vi "Measurement UI.vi"() -> ()   [LabVIEW 2021, in "Load Transient Response_PMIC.lvlib"]
uses:
  Load Transient Response_PMIC.lvlib
panel:
  in  "MeasGraphs":enum32{"LOAD TRANSIENT", "Hidden Controls"}(tab)
  out "LoadCurrentV/STimeGraph":waveform(dbl)(graph) caption="Load Transient"
  out "OutputVoltageV/STimeGraph":waveform(dbl)(graph) caption="Load Transient"
  in  "Load Current v/s Time":string="LOAD CURRENT vs TIME"
  in  "Output Voltage v/s Time":string="LOAD VOLTAGE vs TIME"
  in  "Source resource name":string
  in  "Load resource name":string
  out "dt":dbl
  out "Load voltages":dbl[](array[numeric])
  out "Load currents":dbl[](array[numeric])
  in  "Source transient response":i32(ring)=1042 items=["Slow"=1041, "Normal"=1038, "Fast"=1039, "Custom"=1042]
  in  "Load transient response":i32(ring)=3 items=["Slow"=1041, "Normal"=1038, "Fast"=1039, "Custom"=1042]
  in  "Load current level range":dbl=6.0 caption="CURRENT LEVEL RANGE" format="%#_6pA"
  in  "Load current rising slew rate":dbl=24.0 caption="CURRENT RISING SLEW RATE" format="%#_6pA/us"
  in  "Load current falling slew rate":dbl=24.0 caption="CURRENT FALLING SLEW RATE" format="%#_6pA/us"
  in  "Load configuration":string="Load configuration"
  in  "Source configuration":string="Source configuration"
  in  "Source voltage level":dbl=12.0 caption="VOLTAGE LEVEL" format="%#_6pV"
  in  "Source current limit":dbl=25.0 caption="CURRENT LIMIT" format="%#_6pA"
  in  "PPSResourceName":refnum<k15> caption="RESOURCE NAME"
  in  "Source voltage pole-zero ratio":dbl=2.0 caption="POLE-ZERO RATIO"
  in  "Source voltage gain bandwidth":dbl=2000.0 caption="GAIN BANDWIDTH" format="%#_6pHz"
  in  "Source voltage compensation frequency":dbl=3530.0 caption="COMP. FREQUENCY" format="%#_6pHz"
  in  "Source fast":bool
  in  "Source normal":bool
  in  "Source slow":bool
  in  "Source SourceAdapt":string="Voltage SourceAdapt Parameters"
  in  "Load voltage limit range":dbl=6.0 caption="VOLTAGE LIMIT RANGE" format="%#_6pV"
  in  "Load current set point 1":dbl=4.0 caption="CURRENT SET POINT 1" format="%#_6pA"
  in  "Load current pole-zero ratio":dbl=0.3 caption="POLE-ZERO RATIO"
  in  "Load current gain bandwidth":dbl=14000.0 caption="GAIN BANDWIDTH" format="%#_6pHz"
  in  "Load current compensation frequency":dbl=180000.0 caption="COMP. FREQUENCY" format="%#_6pHz"
  in  "Load sample rate":dbl=1800000.0 caption="SAMPLE RATE" format="%#_6pS/s"
  in  "Load current set point 2":dbl=14.0 caption="CURRENT SET POINT 2" format="%#_6pA"
  in  "ELOADResourceName":refnum<k15> caption="RESOURCE NAME"
  in  "Load fast":bool
  in  "Load normal":bool
  in  "Load slow":bool
  in  "Load SourceAdapt":string="Current SourceAdapt Parameters"
  out "Status":string
  in  "DUT setup time":dbl=1.0 caption="DUT SETUP TIME" format="%#_6ps"
  in  "Level dwell time":dbl=0.001 caption="LEVEL DWELL TIME" format="%#_6ps"
  in  "Measurement settings":string="Measurement settings"
  in  "Nominal output voltage":dbl=3.3 caption="NOMINAL OUTPUT VOLTAGE" format="%#_6pV"
  in  "Mode of operation":T1(ring)=enum."Perform measurement" caption="MODE OF OPERATION"
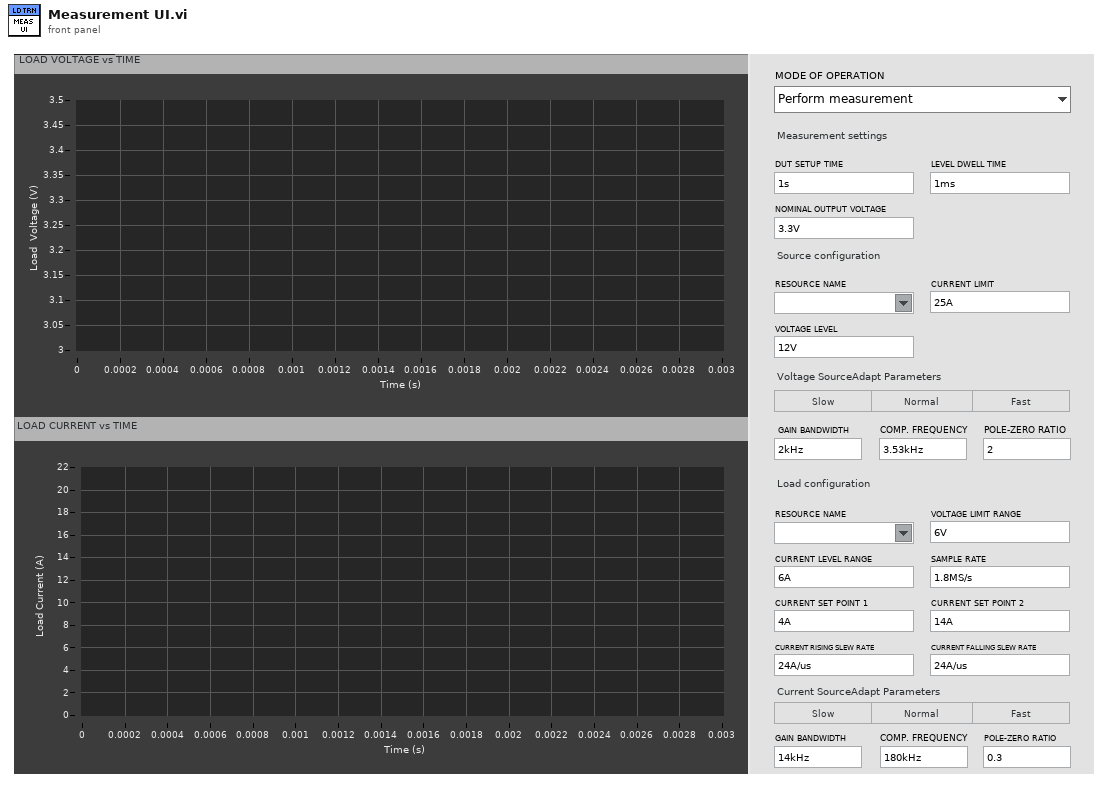
[diagram p1: front panel]
types:
  T1 = enum32{"Power on the DUT", "Perform measurement", "Power off the DUT"}
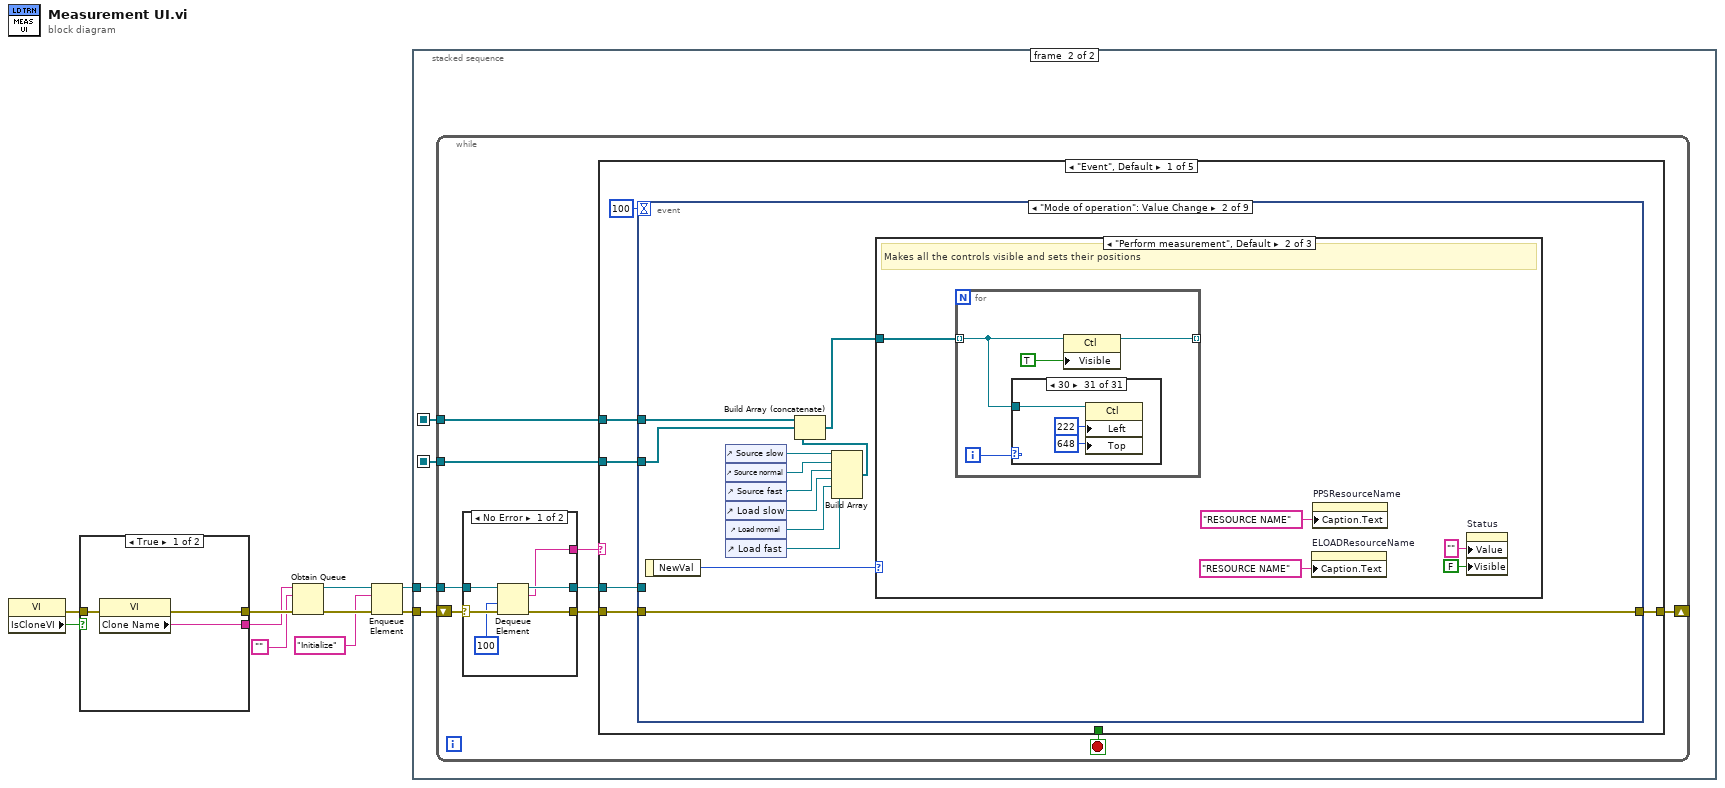
[diagram p0: block diagram]
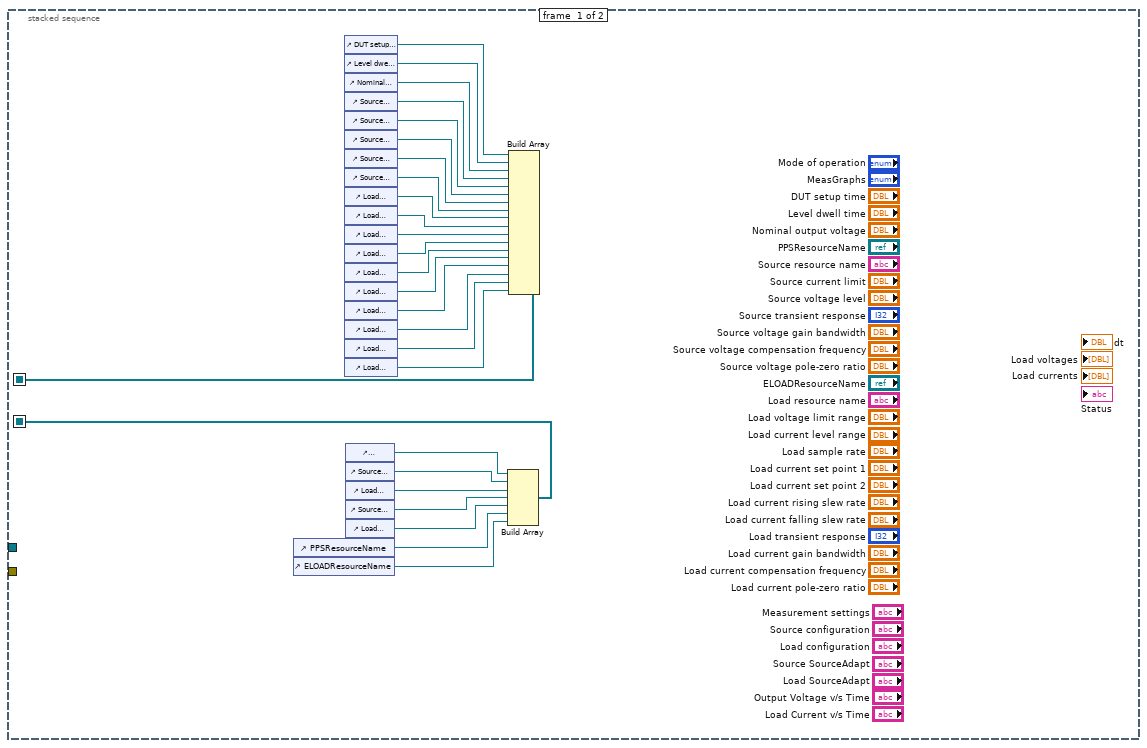
[diagram p2: hidden frame]
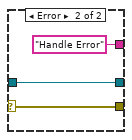
[diagram p3: hidden frame]
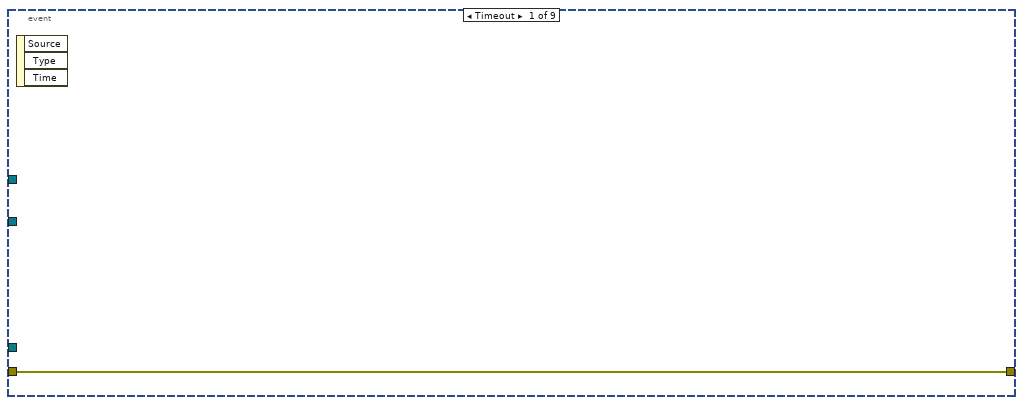
[diagram p4: hidden frame]
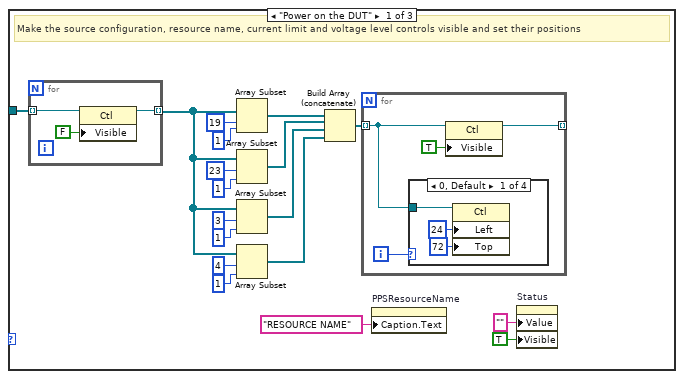
[diagram p5: hidden frame]
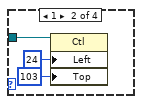
[diagram p6: hidden frame]
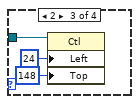
[diagram p7: hidden frame]
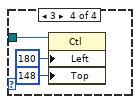
[diagram p8: hidden frame]
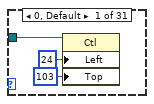
[diagram p9: hidden frame]
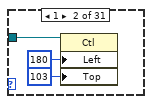
[diagram p10: hidden frame]
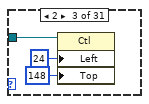
[diagram p11: hidden frame]
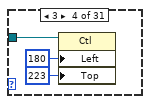
[diagram p12: hidden frame]
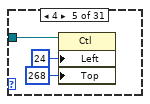
[diagram p13: hidden frame]
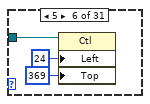
[diagram p14: hidden frame]
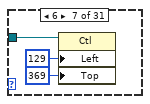
[diagram p15: hidden frame]
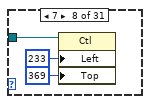
[diagram p16: hidden frame]
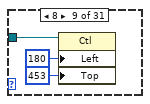
[diagram p17: hidden frame]
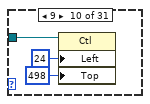
[diagram p18: hidden frame]
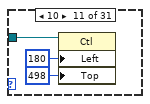
[diagram p19: hidden frame]
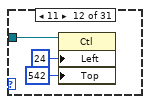
[diagram p20: hidden frame]
diagram:
  n1 = property class="VI"() -> (error out=w1:errorcluster, "IsCloneVI"=w2:bool)  [unwired: 2 in, 1 out]
  n2 = case shown="True" w2 {
    tunnel: [w13 w16] -> w10
    tunnel: [w12 w15] -> w9
    tunnel: w1 -> [w11 w14]
    frame True {
      n3 = property class="VI"(error in=w11) -> (error out=w13:errorcluster, "Clone Name"=w12:string)  [unwired: 1 in, 1 out]
    }
    frame False {
      n4 = property class="VI"(error in=w14) -> (error out=w16:errorcluster, "Name"=w15:string)  [unwired: 1 in, 1 out]
    }
  }
  n5 = Obtain Queue(name (unnamed)=w9, element data type="", error in (no error)=w10) -> (queue out=w6:refnum<queue>, error out=w8:errorcluster)  [unwired: 2 in, 1 out]
  n6 = Enqueue Element(queue=w6, element="Initialize", error in (no error)=w8) -> (queue out=w5:refnum<queue>, error out=w7:errorcluster)  [unwired: 1 in, 1 out]
  n7 = stacked-sequence {
    seq-local: [w25 _] -> [_ w45]
    seq-local: [w26 _] -> [_ w44]
    tunnel: w7 -> [_ w47]
    tunnel: w5 -> [_ w46]
    frame #0 {
      n8 = control-ref of="PPSResourceName"() -> (w29:refnum<vi>)
      n9 = control-ref of="ELOADResourceName"() -> (w30:refnum<vi>)
      n10 = control-ref of="DUT setup time"() -> (w43:refnum<vi>)
      n11 = control-ref of="Level dwell time"() -> (w42:refnum<vi>)
      n12 = control-ref of="Nominal output voltage"() -> (w41:refnum<vi>)
      n13 = control-ref of="Source current limit"() -> (w40:refnum<vi>)
      n14 = control-ref of="Source voltage level"() -> (w39:refnum<vi>)
      n15 = control-ref of="Source voltage gain bandwidth"() -> (w38:refnum<vi>)
      n16 = control-ref of="Source voltage compensation frequency"() -> (w37:refnum<vi>)
      n17 = control-ref of="Source voltage pole-zero ratio"() -> (w36:refnum<vi>)
      n18 = control-ref of="Load voltage limit range"() -> (w35:refnum<vi>)
      n19 = control-ref of="Load current level range"() -> (w20:refnum<vi>)
      n20 = control-ref of="Load sample rate"() -> (w34:refnum<vi>)
      n21 = control-ref of="Load current set point 1"() -> (w33:refnum<vi>)
      n22 = control-ref of="Load current set point 2"() -> (w32:refnum<vi>)
      n23 = control-ref of="Load current rising slew rate"() -> (w19:refnum<vi>)
      n24 = control-ref of="Load current falling slew rate"() -> (w17:refnum<vi>)
      n25 = control-ref of="Load current gain bandwidth"() -> (w18:refnum<vi>)
      n26 = control-ref of="Load current compensation frequency"() -> (w31:refnum<vi>)
      n27 = control-ref of="Load current pole-zero ratio"() -> (w27:refnum<vi>)
      n28 = control-ref of="Measurement settings"() -> (w28:refnum<vi>)
      n29 = control-ref of="Source configuration"() -> (w24:refnum<vi>)
      n30 = control-ref of="Load configuration"() -> (w23:refnum<vi>)
      n31 = control-ref of="Source SourceAdapt"() -> (w22:refnum<vi>)
      n32 = control-ref of="Load SourceAdapt"() -> (w21:refnum<vi>)
      n33 = Build Array(w28, w24, w23, w22, w21, w29, w30) -> (w26:refnum<vi>[])
      n34 = Build Array(w43, w42, w41, w40, w39, w38, w37, w36, w35, w20, w34, w33, w32, w19, w17, w18, w31, w27) -> (w25:refnum<vi>[])
    }
    frame #1 {
      n35 = while {
        shift-right: [w51] -> _
        shift-left: w47 -> [w56]
        tunnel: w46 -> [w54]
        tunnel: w45 -> [w49]
        tunnel: w44 -> [w48]
        stop <- w50 stop-if-true
        n36 = case shown="No Error" w56 {
          selector: w56 -> [w62 w65]
          tunnel: [w61 w65] -> w55
          tunnel: w54 -> [w60 w64]
          tunnel: [w59 w64] -> w53
          tunnel: [w58 "Handle Error"] -> w52
          frame No Error {
            n37 = Dequeue Element(queue=w60, timeout in ms (-1)=100, error in (no error)=w62) -> (queue out=w59:refnum<queue>, element=w58:string, error out=w61:errorcluster)  [unwired: 1 out]
          }
          frame Error {
          }
        }
        n38 = case shown="\"Event\", Default" w52 {
          tunnel: w55 -> [w70 w297 w303 w315 w316]
          tunnel: w53 -> [w68 _ _ w313 _]
          tunnel: [w71 w297 w303 w304 w316] -> w51
          tunnel: [_ FALSE _ TRUE _] -> w50
          tunnel: w49 -> [w67 _ _ w309 _]
          tunnel: w48 -> [w66 _ _ w308 _]
          frame "Event", Default {
            n39 = event shown="[1] \"Mode of operation\": Value Change" {
              selector: _ -> [_ _ _ _ _ _ _ _ _]
              dyn-events: _ -> [_ _ _ _ _ _ _ _ _]
              timeout: 100 -> [_ _ _ _ _ _ _ _ _]
              tunnel: [w72 w80 w246 w248 _ _ _ _ w290] -> w71
              tunnel: w70 -> [w72 w80 w246 w248 _ _ _ _ w291]
              tunnel: w68 -> [_ _ _ _ _ _ _ _ w289]
              tunnel: w67 -> [_ w82 _ _ _ _ _ _ _]
              tunnel: w66 -> [_ w81 _ _ _ _ _ _ _]
              event Timeout {
                n40 = event-data() -> ()  [unwired: 1 in, 3 out]
              }
              event "Mode of operation": Value Change {
                n41 = event-data() -> ("NewVal"=w84:T1)  [unwired: 1 in]
                n42 = control-ref of="Source slow"() -> (w79:refnum<vi>)
                n43 = control-ref of="Source normal"() -> (w78:refnum<vi>)
                n44 = control-ref of="Source fast"() -> (w74:refnum<vi>)
                n45 = control-ref of="Load slow"() -> (w77:refnum<vi>)
                n46 = control-ref of="Load normal"() -> (w76:refnum<vi>)
                n47 = control-ref of="Load fast"() -> (w75:refnum<vi>)
                n48 = Build Array(w79, w78, w74, w77, w76, w75) -> (w73:refnum<vi>[])
                n49 = Build Array (concatenate)(w82, w81, w73) -> (w83:refnum<vi>[])
                n50 = case shown="\"Perform measurement\", Default" w84 {
                  tunnel: w83 -> [w88 w126 w228]
                  frame "Power on the DUT" {
                    # "Make the source configuration, resource name, current limit and voltage level controls visible and set their positions"
                    n51 = for {
                      tunnel: w88 -> [w105] mode=indexing
                      tunnel: [w103] -> w99 mode=indexing
                      n52 = property class="Ctl"(reference=w105, "Visible"=FALSE) -> (reference out=w103:refnum<vi>)  [unwired: 1 in, 1 out]
                    }
                    n53 = Array Subset(array=w99, index=19 ("length"), length=1 ("index")) -> (w97:refnum<vi>[])
                    n54 = Array Subset(array=w99, index=23 ("length"), length=1 ("index")) -> (w98:refnum<vi>[])
                    n55 = Array Subset(array=w99, index=3 ("length"), length=1 ("index")) -> (w100:refnum<vi>[])
                    n56 = Array Subset(array=w99, index=4 ("length"), length=1 ("index")) -> (w102:refnum<vi>[])
                    n57 = Build Array (concatenate)(w97, w98, w100, w102) -> (w101:refnum<vi>[])
                    n58 = for {
                      tunnel: [w108] -> _ mode=indexing
                      tunnel: w101 -> [w106] mode=indexing
                      i -> [w107]
                      n59 = case shown="0, Default" w107 {
                        tunnel: w106 -> [w112 w115 w118 w121]
                        frame 0, Default {
                          n60 = property class="Ctl"(reference=w112, "Left"=24 ("Position:Left"), "Top"=72 ("Position:Top")) -> ()  [unwired: 1 in, 2 out]
                        }
                        frame 1 {
                          n61 = property class="Ctl"(reference=w115, "Left"=24 ("Position:Left"), "Top"=103 ("Position:Top")) -> ()  [unwired: 1 in, 2 out]
                        }
                        frame 2 {
                          n62 = property class="Ctl"(reference=w118, "Left"=24 ("Position:Left"), "Top"=148 ("Position:Top")) -> ()  [unwired: 1 in, 2 out]
                        }
                        frame 3 {
                          n63 = property class="Ctl"(reference=w121, "Left"=180 ("Position:Left"), "Top"=148 ("Position:Top")) -> ()  [unwired: 1 in, 2 out]
                        }
                      }
                      n64 = property class="Ctl"(reference=w106, "Visible"=TRUE) -> (reference out=w108:refnum<vi>)  [unwired: 1 in, 1 out]
                    }
                    n65 = property on="PPSResourceName" class="IVIName"("Caption.Text"="RESOURCE NAME") -> ()  [unwired: 2 in, 2 out]
                    n66 = property on="Status" class="Str"("Value"="" ("Status"), "Visible"=TRUE) -> ()  [unwired: 2 in, 2 out]
                  }
                  frame "Perform measurement", Default {
                    # "Makes all the controls visible and sets their positions"
                    n67 = for {
                      tunnel: w126 -> [w127] mode=indexing
                      tunnel: [w129] -> _ mode=indexing
                      i -> [w128]
                      n68 = case shown="30" w128 {
                        tunnel: w127 -> [w133 w136 w139 w142 w145 w148 w151 w154 w157 w160 w163 w166 w169 w172 w175 w178 w181 w184 w187 w188 w191 w194 w197 w200 w203 w206 w209 w212 w216 w218 w221]
                        frame 0, Default {
                          n69 = property class="Ctl"(reference=w133, "Left"=24 ("Position:Left"), "Top"=103 ("Position:Top")) -> ()  [unwired: 1 in, 2 out]
                        }
                        frame 1 {
                          n70 = property class="Ctl"(reference=w136, "Left"=180 ("Position:Left"), "Top"=103 ("Position:Top")) -> ()  [unwired: 1 in, 2 out]
                        }
                        frame 2 {
                          n71 = property class="Ctl"(reference=w139, "Left"=24 ("Position:Left"), "Top"=148 ("Position:Top")) -> ()  [unwired: 1 in, 2 out]
                        }
                        frame 3 {
                          n72 = property class="Ctl"(reference=w142, "Left"=180 ("Position:Left"), "Top"=223 ("Position:Top")) -> ()  [unwired: 1 in, 2 out]
                        }
                        frame 4 {
                          n73 = property class="Ctl"(reference=w145, "Left"=24 ("Position:Left"), "Top"=268 ("Position:Top")) -> ()  [unwired: 1 in, 2 out]
                        }
                        frame 5 {
                          n74 = property class="Ctl"(reference=w148, "Left"=24 ("Position:Left"), "Top"=369 ("Position:Top")) -> ()  [unwired: 1 in, 2 out]
                        }
                        frame 6 {
                          n75 = property class="Ctl"(reference=w151, "Left"=129 ("Position:Left"), "Top"=369 ("Position:Top")) -> ()  [unwired: 1 in, 2 out]
                        }
                        frame 7 {
                          n76 = property class="Ctl"(reference=w154, "Left"=233 ("Position:Left"), "Top"=369 ("Position:Top")) -> ()  [unwired: 1 in, 2 out]
                        }
                        frame 8 {
                          n77 = property class="Ctl"(reference=w157, "Left"=180 ("Position:Left"), "Top"=453 ("Position:Top")) -> ()  [unwired: 1 in, 2 out]
                        }
                        frame 9 {
                          n78 = property class="Ctl"(reference=w160, "Left"=24 ("Position:Left"), "Top"=498 ("Position:Top")) -> ()  [unwired: 1 in, 2 out]
                        }
                        frame 10 {
                          n79 = property class="Ctl"(reference=w163, "Left"=180 ("Position:Left"), "Top"=498 ("Position:Top")) -> ()  [unwired: 1 in, 2 out]
                        }
                        frame 11 {
                          n80 = property class="Ctl"(reference=w166, "Left"=24 ("Position:Left"), "Top"=542 ("Position:Top")) -> ()  [unwired: 1 in, 2 out]
                        }
                        frame 12 {
                          n81 = property class="Ctl"(reference=w169, "Left"=180 ("Position:Left"), "Top"=542 ("Position:Top")) -> ()  [unwired: 1 in, 2 out]
                        }
                        frame 13 {
                          n82 = property class="Ctl"(reference=w172, "Left"=24 ("Position:Left"), "Top"=586 ("Position:Top")) -> ()  [unwired: 1 in, 2 out]
                        }
                        frame 14 {
                          n83 = property class="Ctl"(reference=w175, "Left"=180 ("Position:Left"), "Top"=586 ("Position:Top")) -> ()  [unwired: 1 in, 2 out]
                        }
                        frame 15 {
                          n84 = property class="Ctl"(reference=w178, "Left"=24 ("Position:Left"), "Top"=677 ("Position:Top")) -> ()  [unwired: 1 in, 2 out]
                        }
                        frame 16 {
                          n85 = property class="Ctl"(reference=w181, "Left"=129 ("Position:Left"), "Top"=677 ("Position:Top")) -> ()  [unwired: 1 in, 2 out]
                        }
                        frame 17 {
                          n86 = property class="Ctl"(reference=w184, "Left"=233 ("Position:Left"), "Top"=677 ("Position:Top")) -> ()  [unwired: 1 in, 2 out]
                        }
                        frame 18 {
                          n87 = property class="Ctl"(reference=w187, "Left"=24 ("Position:Left"), "Top"=72 ("Position:Top")) -> ()  [unwired: 1 in, 2 out]
                        }
                        frame 19 {
                          n88 = property class="Ctl"(reference=w188, "Left"=24 ("Position:Left"), "Top"=192 ("Position:Top")) -> ()  [unwired: 1 in, 2 out]
                        }
                        frame 20 {
                          n89 = property class="Ctl"(reference=w191, "Left"=24 ("Position:Left"), "Top"=420 ("Position:Top")) -> ()  [unwired: 1 in, 2 out]
                        }
                        frame 21 {
                          n90 = property class="Ctl"(reference=w194, "Left"=24 ("Position:Left"), "Top"=312 ("Position:Top")) -> ()  [unwired: 1 in, 2 out]
                        }
                        frame 22 {
                          n91 = property class="Ctl"(reference=w197, "Left"=24 ("Position:Left"), "Top"=628 ("Position:Top")) -> ()  [unwired: 1 in, 2 out]
                        }
                        frame 23 {
                          n92 = property class="Ctl"(reference=w200, "Left"=24 ("Position:Left"), "Top"=223 ("Position:Top")) -> ()  [unwired: 1 in, 2 out]
                        }
                        frame 24 {
                          n93 = property class="Ctl"(reference=w203, "Left"=24 ("Position:Left"), "Top"=453 ("Position:Top")) -> ()  [unwired: 1 in, 2 out]
                        }
                        frame 25 {
                          n94 = property class="Ctl"(reference=w206, "Left"=24 ("Position:Left"), "Top"=336 ("Position:Top")) -> ()  [unwired: 1 in, 2 out]
                        }
                        frame 26 {
                          n95 = property class="Ctl"(reference=w209, "Left"=121 ("Position:Left"), "Top"=336 ("Position:Top")) -> ()  [unwired: 1 in, 2 out]
                        }
                        frame 27 {
                          n96 = property class="Ctl"(reference=w212, "Left"=222 ("Position:Left"), "Top"=336 ("Position:Top")) -> ()  [unwired: 1 in, 2 out]
                        }
                        frame 28 {
                          n97 = property class="Ctl"(reference=w216, "Left"=24 ("Position:Left"), "Top"=648 ("Position:Top")) -> ()  [unwired: 1 in, 2 out]
                        }
                        frame 29 {
                          n98 = property class="Ctl"(reference=w218, "Left"=121 ("Position:Left"), "Top"=648 ("Position:Top")) -> ()  [unwired: 1 in, 2 out]
                        }
                        frame 30 {
                          n99 = property class="Ctl"(reference=w221, "Left"=222 ("Position:Left"), "Top"=648 ("Position:Top")) -> ()  [unwired: 1 in, 2 out]
                        }
                      }
                      n100 = property class="Ctl"(reference=w127, "Visible"=TRUE) -> (reference out=w129:refnum<vi>)  [unwired: 1 in, 1 out]
                    }
                    n101 = property on="ELOADResourceName" class="IVIName"("Caption.Text"="RESOURCE NAME") -> ()  [unwired: 2 in, 2 out]
                    n102 = property on="PPSResourceName" class="IVIName"("Caption.Text"="RESOURCE NAME") -> ()  [unwired: 2 in, 2 out]
                    n103 = property on="Status" class="Str"("Value"="" ("Operation"), "Visible"=FALSE) -> ()  [unwired: 2 in, 2 out]
                  }
                  frame "Power off the DUT" {
                    # "Makes only the Source and Load Resource Name controls visible and sets their positions"
                    n104 = for {
                      tunnel: w228 -> [w234] mode=indexing
                      tunnel: [w233] -> w232 mode=indexing
                      n105 = property class="Ctl"(reference=w234, "Visible"=FALSE) -> (reference out=w233:refnum<vi>)  [unwired: 1 in, 1 out]
                    }
                    n106 = Array Subset(array=w232, index=20 ("length"), length=2 ("index")) -> (w231:refnum<vi>[])
                    n107 = for {
                      tunnel: w231 -> [w236] mode=indexing
                      tunnel: [w238] -> _ mode=indexing
                      i -> [w237]
                      n108 = case shown="1" w237 {
                        tunnel: w236 -> [w242 w245]
                        frame 0, Default {
                          n109 = property class="Ctl"(reference=w242, "Left"=24 ("Position:Left"), "Top"=72 ("Position:Top")) -> ()  [unwired: 1 in, 2 out]
                        }
                        frame 1 {
                          n110 = property class="Ctl"(reference=w245, "Left"=24 ("Position:Left"), "Top"=117 ("Position:Top")) -> ()  [unwired: 1 in, 2 out]
                        }
                      }
                      n111 = property class="Ctl"(reference=w236, "Visible"=TRUE) -> (reference out=w238:refnum<vi>)  [unwired: 1 in, 1 out]
                    }
                    n112 = property on="ELOADResourceName" class="IVIName"("Caption.Text"="LOAD RESOURCE NAME") -> ()  [unwired: 2 in, 2 out]
                    n113 = property on="PPSResourceName" class="IVIName"("Caption.Text"="SOURCE RESOURCE NAME") -> ()  [unwired: 2 in, 2 out]
                    n114 = property on="Status" class="Str"("Value"="" ("Status"), "Visible"=TRUE) -> ()  [unwired: 2 in, 2 out]
                  }
                }
              }
              event "PPSResourceName": Value Change {
                n115 = event-data() -> ()  [unwired: 1 in, 6 out]
                n116 = property on="PPSResourceName" class="IVIName"() -> ("Value"=w247:refnum<k15>)  [unwired: 2 in, 2 out]
                n117 = property on="Source resource name" class="Str"("Value"=w247) -> ()  [unwired: 2 in, 2 out]
              }
              event "ELOADResourceName": Value Change {
                n118 = event-data() -> ()  [unwired: 1 in, 6 out]
                n119 = property on="ELOADResourceName" class="IVIName"() -> ("Value"=w249:refnum<k15>)  [unwired: 2 in, 2 out]
                n120 = property on="Load resource name" class="Str"("Value"=w249) -> ()  [unwired: 2 in, 2 out]
              }
              event "Source slow", "Source normal", "Source fast": Value Change {
                n121 = event-data() -> ("CtlRef"=w255:refnum<vi>)  [unwired: 1 in]
                n122 = property class="Bool"(reference=w255) -> ("Label.Text"=w254:string)  [unwired: 1 in, 2 out]
                n123 = case shown="\"Source fast\"" w254 {
                  tunnel: [w259 w263 w267] -> w253
                  tunnel: [500.0 ("Source voltage gain bandwidth") 2000.0 ("Source voltage gain bandwidth") 4000.0 ("Source voltage gain bandwidth")] -> w252
                  tunnel: [1120.0 ("Source voltage compensation frequency") 3530.0 ("Source voltage compensation frequency") 11300.0 ("Source voltage compensation frequency")] -> w251
                  tunnel: [5.0 ("Source voltage pole-zero ratio") 2.0 ("Source voltage pole-zero ratio") 1.5 ("Source voltage pole-zero ratio")] -> w250
                  frame "Source slow" {
                    w259 = 1041 items=["Slow"=1041, "Normal"=1038, "Fast"=1039, "Custom"=1042] ("Source transient response")
                  }
                  frame "Source normal", Default {
                    w263 = 1038 items=["Slow"=1041, "Normal"=1038, "Fast"=1039, "Custom"=1042] ("Source transient response")
                  }
                  frame "Source fast" {
                    w267 = 1039 items=["Slow"=1041, "Normal"=1038, "Fast"=1039, "Custom"=1042] ("Source transient response")
                  }
                }
                n124 = property on="Source transient response" class="Ring (strict)"("Value"=w253) -> ()  [unwired: 2 in, 2 out]
                n125 = property on="Source voltage gain bandwidth" class="DigNum (strict)"("Value"=w252) -> ()  [unwired: 2 in, 2 out]
                n126 = property on="Source voltage compensation frequency" class="DigNum (strict)"("Value"=w251) -> ()  [unwired: 2 in, 2 out]
                n127 = property on="Source voltage pole-zero ratio" class="DigNum (strict)"("Value"=w250) -> ()  [unwired: 2 in, 2 out]
              }
              event "Source voltage gain bandwidth", "Source voltage compensation frequency", "Source voltage pole-zero ratio": Value Change {
                w268 = 1042 items=["Slow"=1041, "Normal"=1038, "Fast"=1039, "Custom"=1042] ("Source transient response")
                n128 = event-data() -> ()  [unwired: 1 in, 1 out]
                n129 = property on="Source transient response" class="Ring (strict)"("Value"=w268) -> ()  [unwired: 2 in, 2 out]
              }
              event "Load slow", "Load normal", "Load fast": Value Change {
                n130 = event-data() -> ("CtlRef"=w273:refnum<vi>)  [unwired: 1 in]
                n131 = property class="Bool"(reference=w273) -> ("Label.Text"=w274:string)  [unwired: 1 in, 2 out]
                n132 = case shown="\"Load normal\", Default" w274 {
                  tunnel: [w278 w282 w286] -> w272
                  tunnel: [300.0 ("Load current gain bandwidth") 4000.0 ("Load current gain bandwidth") 14000.0 ("Load current gain bandwidth")] -> w271
                  tunnel: [1500.0 ("Load current compensation frequency") 25000.0 ("Load current compensation frequency") 180000.0 ("Load current compensation frequency")] -> w270
                  tunnel: [0.3 ("Load current pole-zero ratio") 6.0 ("Load current pole-zero ratio") 0.3 ("Load current pole-zero ratio")] -> w269
                  frame "Load slow" {
                    w278 = 1041 items=["Slow"=1041, "Normal"=1038, "Fast"=1039, "Custom"=1042] ("Source transient response")
                  }
                  frame "Load normal", Default {
                    w282 = 1038 items=["Slow"=1041, "Normal"=1038, "Fast"=1039, "Custom"=1042] ("Source transient response")
                  }
                  frame "Load fast" {
                    w286 = 1039 items=["Slow"=1041, "Normal"=1038, "Fast"=1039, "Custom"=1042] ("Source transient response")
                  }
                }
                n133 = property on="Load transient response" class="Ring (strict)"("Value"=w272) -> ()  [unwired: 2 in, 2 out]
                n134 = property on="Load current gain bandwidth" class="DigNum (strict)"("Value"=w271) -> ()  [unwired: 2 in, 2 out]
                n135 = property on="Load current compensation frequency" class="DigNum (strict)"("Value"=w270) -> ()  [unwired: 2 in, 2 out]
                n136 = property on="Load current pole-zero ratio" class="DigNum (strict)"("Value"=w269) -> ()  [unwired: 2 in, 2 out]
              }
              event "Load current gain bandwidth", "Load current compensation frequency", "Load current pole-zero ratio": Value Change {
                w287 = 1042 items=["Slow"=1041, "Normal"=1038, "Fast"=1039, "Custom"=1042] ("Load transient response")
                n137 = event-data() -> ()  [unwired: 1 in, 1 out]
                n138 = property on="Load transient response" class="Ring (strict)"("Value"=w287) -> ()  [unwired: 2 in, 2 out]
              }
              event Panel Close? {
                n139 = event-data() -> ()  [unwired: 1 in, 4 out]
                n140 = Enqueue Element(queue=w289, element="Exit", error in (no error)=w291) -> (error out=w290:errorcluster)  [unwired: 1 in, 2 out]
                n141 = event-data("Discard?"=TRUE) -> ()  [unwired: 1 in, 1 out]
              }
            }
          }
          frame "Initialize" {
            w294 = 2 ("Palette:Active Tool")
            w295 = "<Select Device>"
            n142 = property on="OutputVoltageV/STimeGraph" class="WFGraph (strict)"("ActPaletteTool"=w294) -> ()  [unwired: 2 in, 2 out]
            n143 = property on="PPSResourceName" class="IVIName"("Value"=w295) -> ()  [unwired: 2 in, 2 out]
            n144 = property on="ELOADResourceName" class="IVIName"("Value"=w295) -> ()  [unwired: 2 in, 2 out]
            n145 = property on="LoadCurrentV/STimeGraph" class="WFGraph (strict)"("ActPaletteTool"=w294) -> ()  [unwired: 2 in, 2 out]
            n146 = property on="Status" class="Str"("Visible"=FALSE) -> ()  [unwired: 2 in, 2 out]
          }
          frame "Post UI Update" {
            # "This case will be triggered, after framework updates the User interface with result values."
            n147 = local read "Load voltages"() -> (w300:dbl[])
            n148 = local read "Load currents"() -> (w299:dbl[])
            n149 = local read "dt"() -> (w298:dbl)
            n150 = Bundle By Name("Y"=w300, "dt"=w298) -> (→"OutputVoltageV/STimeGraph":waveform(dbl))  [unwired: 1 in]
            n151 = Bundle By Name("dt"=w298, "Y"=w299) -> (→"LoadCurrentV/STimeGraph":waveform(dbl))  [unwired: 1 in]
          }
          frame "Exit" {
            # "This case is triggered to close the User Interface from framework"
            n152 = Build Array (concatenate)(w309, w308) -> (w307:refnum<vi>[])
            n153 = Close Reference(reference=w307) -> (error out=w305:errorcluster)  [unwired: 1 in]
            n154 = Flush Queue(queue=w313, error in (no error)=w315) -> (queue out=w312:refnum<queue>, error out=w311:errorcluster)  [unwired: 1 out]
            n155 = Release Queue(queue=w312, force destroy? (F)=TRUE, error in (no error)=w311) -> (error out=w306:errorcluster)  [unwired: 2 out]
            n156 = Merge Errors(w305, w306) -> (w304:errorcluster)
          }
          frame "Handle Error" {
          }
        }
      }
    }
  }
